vi "Open Waveform Sessions.vi"(8 "error in":errorcluster, 11 "Async State Vars":T1) -> (0 "error out":errorcluster, 3 "Async State Vars out":T1)   [LabVIEW 2015, in "Waveform-Processing-Custom-Device Engine.lvlib"]
uses:
  Waveform-Processing-Custom-Device Engine.lvlib
  Types/Async State Vars.ctl
  Types/Async FIFOs.ctl
  <vilib>/NI Veristand/Custom Device Waveform API/Single Waveform Read (DBL)/Single Waveform Read (DBL).lvclass
  <vilib>/NI Veristand/Custom Device Waveform API/Single Waveform Write (DBL)/Single Waveform Write (DBL).lvclass
  <vilib>/NI Veristand/Custom Device API/Waveform Data Reference.ctl
  <vilib>/NI Veristand/Custom Device Waveform API/Single Waveform Read (DBL)/NI VeriStand - Open Single Waveform Read Session (DBL).vi
  <vilib>/NI Veristand/Custom Device Waveform API/Single Waveform Write (DBL)/NI VeriStand - Open Single Waveform Write Session (DBL).vi
  <vilib>/NI Veristand/Custom Device Waveform API/NI_VS Custom Device Waveform API.lvlib
  <vilib>/NI VeriStand/Custom Device API/Custom Device API.lvlib
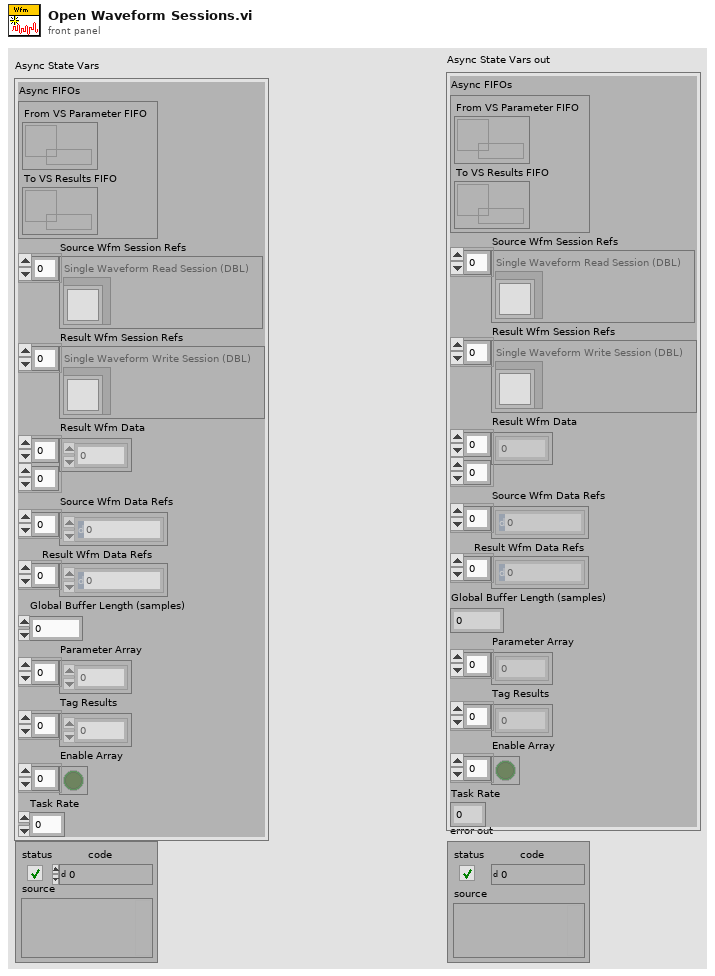
[diagram p1: front panel]
types:
  T1 = typedef "Waveform-Processing-Custom-Device Engine.lvlib/Async State Vars.ctl" = cluster{"Async FIFOs":T2, "Source Wfm Session Refs":refnum<class "Single Waveform Read (DBL).lvclass">[], "Result Wfm Session Refs":refnum<class "Single Waveform Write (DBL).lvclass">[], "Result Wfm Data":dbl[][], "Source Wfm Data Refs":T3[], "Result Wfm Data Refs":T3[], "Global Buffer Length (samples)":dbl, "Parameter Array":dbl[], "Tag Results":dbl[], "Enable Array":bool[], "Task Rate":dbl}
  T2 = typedef "Waveform-Processing-Custom-Device Engine.lvlib/Async FIFOs.ctl" = cluster{"From VS Parameter FIFO":refnum<k33>, "To VS Results FIFO":refnum<k33>}
  T3 = typedef "Custom Device API.lvlib/Waveform Data Reference.ctl" = i32
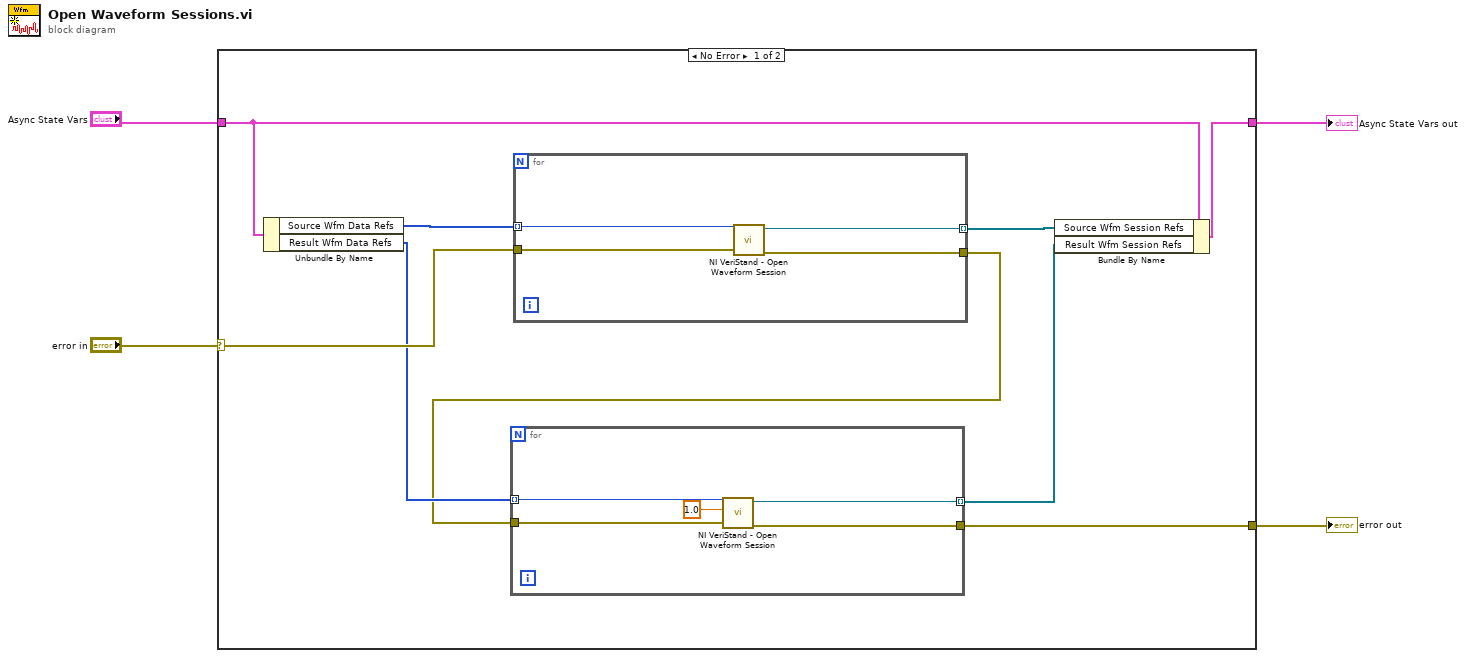
[diagram p0: block diagram]
diagram:
  n1 = case shown="No Error" "error in" {
    selector: "error in" -> [w10 w24]
    tunnel: [w5 w24] -> w3
    tunnel: "Async State Vars" -> [w9 w23]
    tunnel: [w11 w23] -> w1
    frame No Error {
      n2 = Unbundle By Name(w9) -> ("Source Wfm Data Refs"=w13:T3[], "Result Wfm Data Refs"=w8:T3[])
      n3 = for {
        tunnel: [w22] -> w7
        tunnel: w13 -> [w20] mode=indexing
        tunnel: [w21] -> w12 mode=indexing
        tunnel: w10 -> [w19]
        n4 = call-poly <vilib>:"NI VeriStand - Open Waveform Session.vi"("error in (no error)"=w19, "DBL Waveform Data Reference"=w20) -> ("error out"=w22:errorcluster, "Single Waveform Read Session (DBL)"=w21:refnum<class "Single Waveform Read (DBL).lvclass">)  [unwired: 8 in]
      }
      n5 = for {
        tunnel: [w18] -> w5
        tunnel: w8 -> [w16] mode=indexing
        tunnel: [w17] -> w6 mode=indexing
        tunnel: w7 -> [w15]
        n6 = call-poly <vilib>:"NI VeriStand - Open Waveform Session.vi"("error in (no error)"=w15, "dt"=1.0, "DBL Waveform Data Reference"=w16) -> ("error out"=w18:errorcluster, "Single Waveform Write Session (DBL)"=w17:refnum<class "Single Waveform Write (DBL).lvclass">)  [unwired: 7 in]
      }
      n7 = Bundle By Name(cluster=w9, "Source Wfm Session Refs"=w12, "Result Wfm Session Refs"=w6) -> (w11:T1)
    }
    frame Error {
    }
  }
  "error out" <- w3
  "Async State Vars out" <- w1
